vi "_Read ItemArray.vi"(6 "Config Path":path, 7 "Section Prefix":string="CSMAPI", 8 "Error In":errorcluster caption="Error in (no error)", 11 "Section":string) -> (0 "Error Out":errorcluster, 3 "Array":string[](array[string]))   [LabVIEW 2017, in "CSM-Helper API with lvcsm Support.lvlib"]
uses:
  CSM-Helper API with lvcsm Support.lvlib
  <vilib>/Utility/config.llb/Read Key (String).vi
  <vilib>/Utility/config.llb/NI_LVConfig.lvlib
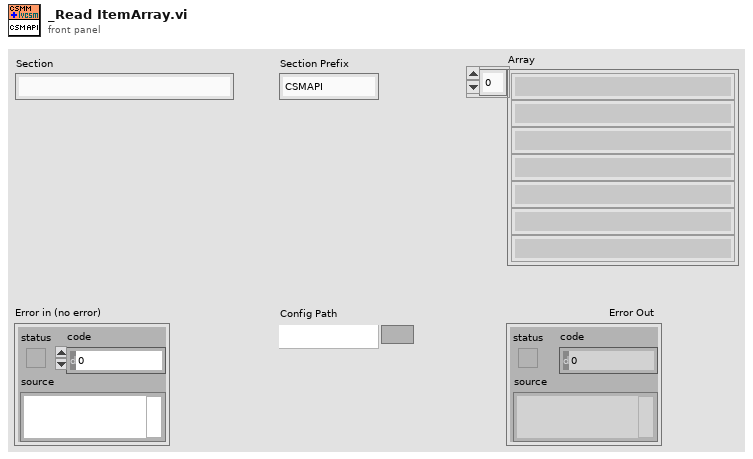
[diagram p1: front panel]
types:
  T1 = typedef "NI_LVConfig.lvlib/Config Data RefNum.ctl" = refnum<k1>
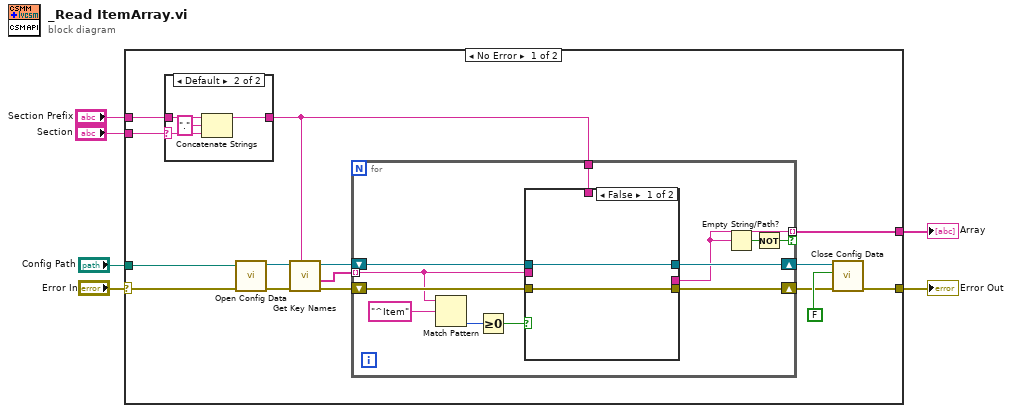
[diagram p0: block diagram]
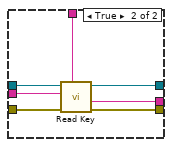
[diagram p2: hidden frame]
diagram:
  n1 = case shown="No Error" "Error In" {
    selector: "Error In" -> [w19 w48]
    tunnel: [w20 w48] -> w5
    tunnel: "Config Path" -> [w21 _]
    tunnel: [w8 _] -> w3
    tunnel: "Section" -> [w15 _]
    tunnel: "Section Prefix" -> [w7 _]
    frame No Error {
      n2 = case shown="Default" w15 {
        selector: w15 -> [_ w45]
        tunnel: w7 -> [w43 w47]
        tunnel: [w43 w46] -> w9
        frame "" {
        }
        frame Default {
          n3 = Concatenate Strings(w47, "." ("string"), w45) -> (w46:string)
        }
      }
      n4 = call <vilib>:"Open Config Data.vi"("error in (no error)"=w19, "configuration file path"=w21) -> ("error out"=w16:errorcluster, "refnum"=w18:T1)  [unwired: 7 in, 1 out]
      n5 = call <vilib>:"Get Key Names.vi"("section"=w9, "error in (no error)"=w16, "refnum"=w18) -> ("error out"=w14:errorcluster, "key names"=w10:string[], "refnum out"=w13:T1)  [unwired: 5 in, 1 out]
      n6 = for {
        tunnel: w10 -> [w25] mode=indexing
        tunnel: w9 -> [w29]
        shift-right: [w31] -> w12
        shift-left: w14 -> [w33]
        shift-right: [w30] -> w11
        shift-left: w13 -> [w32]
        tunnel: [w28] -> w8 mode=indexing if=w26
        n7 = Match Pattern(string=w25, regular expression="^Item") -> (offset past match=w23:i32)  [unwired: 1 in, 3 out]
        n8 = Greater Or Equal To 0?(x=w23) -> (x >= 0?=w22:bool)
        n9 = case shown="False" w22 {
          tunnel: w33 -> [w35 w42]
          tunnel: w32 -> [w34 w41]
          tunnel: [w35 w40] -> w31
          tunnel: [w34 w39] -> w30
          tunnel: w29 -> [_ w38]
          tunnel: [_ w37] -> w28
          tunnel: w25 -> [_ w36]
          frame False {
          }
          frame True {
            n10 = call-poly <vilib>:"Read Key.vi"("section"=w38, "error in (no error)"=w42, "key"=w36, "refnum"=w41) -> ("error out"=w40:errorcluster, "value"=w37:string, "refnum out"=w39:T1)  [unwired: 4 in, 1 out]
          }
        }
        n11 = Empty String/Path?(string/path=w28) -> (empty?=w27:bool)
        n12 = Not(x=w27) -> (.not. x?=w26:bool)
      }
      n13 = call <vilib>:"Close Config Data.vi"("error in (no error)"=w12, "write file if changed (T)"=FALSE, "refnum"=w11) -> ("error out"=w20:errorcluster)  [unwired: 7 in, 1 out]
    }
    frame Error {
    }
  }
  "Error Out" <- w5
  "Array" <- w3
